vi "Parse Xml Recursively.vi"(7 "Parent":string, 8 "error in":errorcluster, 9 "XML File Path":path, 10 "DOM document in":refnum<k20>, 11 "VI Data":T1[](array[typedef])) -> (0 "error out":errorcluster, 3 "VI Data out":T1[](array[typedef]))   [LabVIEW 2020, in "VI Properties Editor.lvlib"]
uses:
  VI Properties Editor.lvlib
  CTLs/XPath Get Attribute.ctl
  <vilib>/picture/picture.llb/imagedata.ctl
  CTLs/VI Properties.ctl
  CTLs/Control Properties.ctl
  CTLs/VI Data.ctl
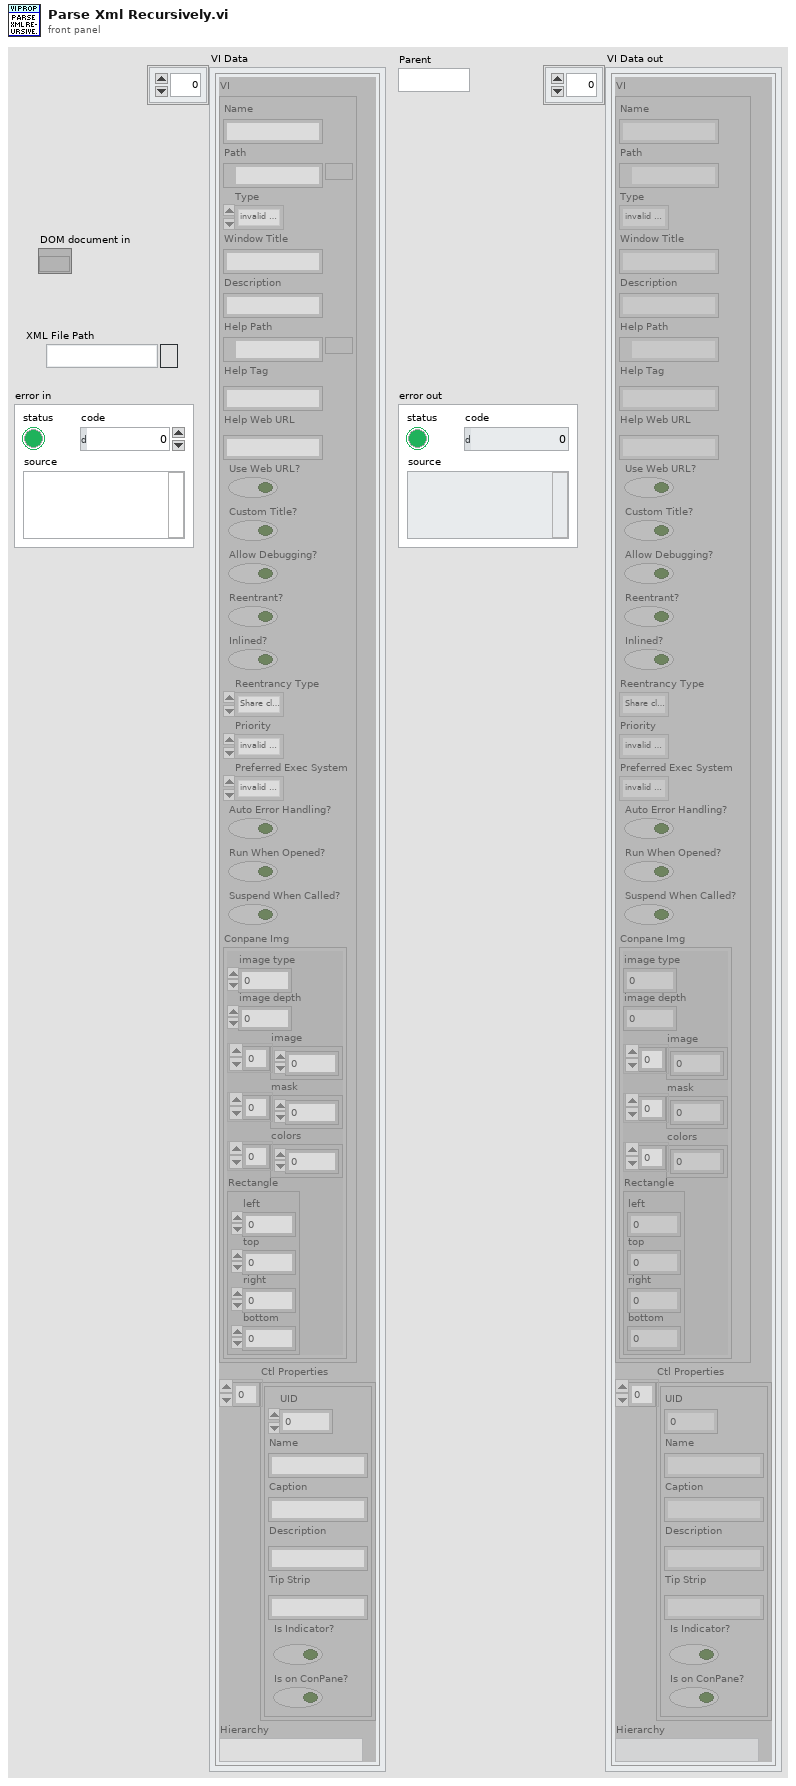
[diagram p1: front panel]
types:
  T1 = typedef "VI Properties Editor.lvlib/VI Data.ctl" = cluster{"VI":T2, "Ctl Properties":T4[], "Hierarchy":string}
  T2 = typedef "VI Properties Editor.lvlib/VI Properties.ctl" = cluster{"Name":string, "Path":path, "Type":enum32{"invalid VI type", "Standard VI", "Control VI", "Global VI", "Polymorphic VI", "Configuration VI", "SubSystem", "Facade VI", "Method VI", "Statechart Diagram VI"}, "Window Title":string, "Description":string, "Help Path":path, "Help Tag":string, "Help Web URL":string, "Use Web URL?":bool, "Custom Title?":bool, "Allow Debugging?":bool, "Reentrant?":bool, "Inlined?":bool, "Reentrancy Type":enum16{"Share clones between instances", "Preallocate clone for each instance"}, "Priority":enum32{"invalid priority", "background priority", "normal priority", "above normal priority", "high priority", "time critical priority", "subroutine"}, "Preferred Exec System":enum32{"invalid execution system", "user interface", "standard", "instrument i/o", "data acquisition", "other 1", "other 2", "same as caller"}, "Auto Error Handling?":bool, "Run When Opened?":bool, "Suspend When Called?":bool, "Conpane Img":T3}
  T3 = typedef "imagedata.ctl" = cluster{"image type":i32, "image depth":i32, "image":u8[], "mask":u8[], "colors":u32[], "Rectangle":cluster{"left":i16, "top":i16, "right":i16, "bottom":i16}}
  T4 = typedef "VI Properties Editor.lvlib/Control Properties.ctl" = cluster{"UID":i32, "Name":string, "Caption":string, "Description":string, "Tip Strip":string, "Is Indicator?":bool, "Is on ConPane?":bool}
  T5 = typedef "VI Properties Editor.lvlib/XPath Get Attribute.ctl" = enum16{"Item[@Type='VI']/@URL", "Item[@Type='LVClass']/@URL", "Item[@Type='Library']/@URL", "@Name"}
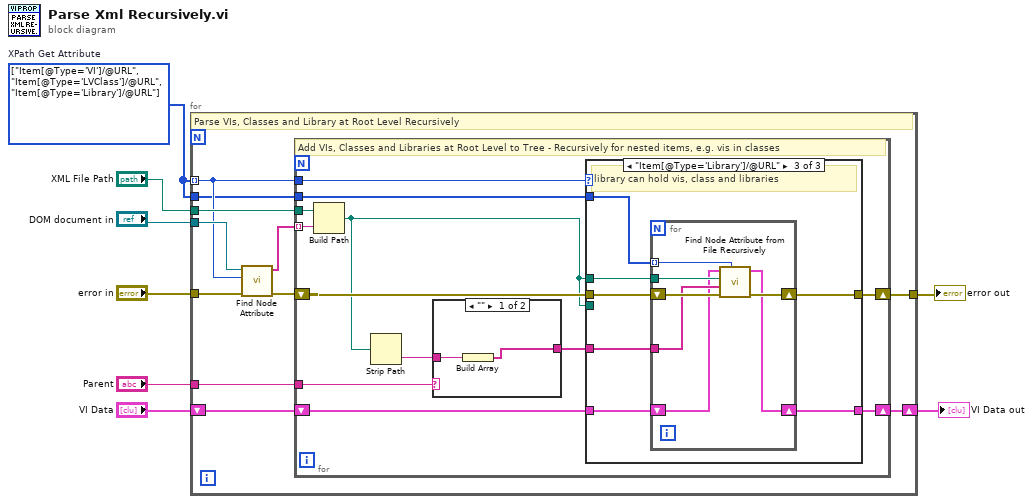
[diagram p0: block diagram]
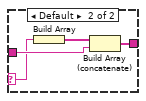
[diagram p2: hidden frame]
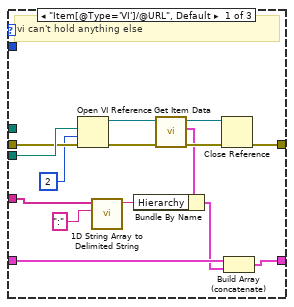
[diagram p3: hidden frame]
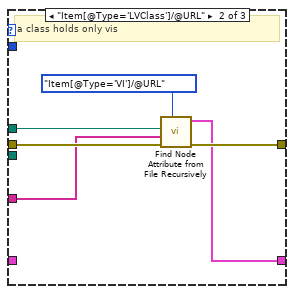
[diagram p4: hidden frame]
diagram:
  w5 = T5[] [enum."Item[@Type='VI']/@URL", enum."Item[@Type='LVClass']/@URL", enum."Item[@Type='Library']/@URL"] items=["Item[@Type='VI']/@URL", "Item[@Type='LVClass']/@URL", "Item[@Type='Library']/@URL", "@Name"]  # XPath Get Attribute
  n1 = for {
    tunnel: "XML File Path" -> [w18]
    tunnel: [w17] -> w6
    tunnel: "DOM document in" -> [w15]
    tunnel: "error in" -> [w14]
    tunnel: "Parent" -> [w13]
    shift-right: [w11] -> w1
    shift-left: "VI Data" -> [w12]
    tunnel: w5 -> [w10] mode=indexing
    tunnel: w5 -> [w9]
    # "Parse VIs, Classes and Library at Root Level Recursively"
    n2 = call "Find Node Attribute.vi"("error in"=w14, "XPath"=w10, "Node"=w15) -> ("error out"=w16:errorcluster, "Attribute"=w19:string[])  [unwired: 7 in]
    n3 = for {
      shift-right: [w31] -> w17
      shift-left: w16 -> [w27]
      tunnel: w10 -> [w28]
      tunnel: w18 -> [w29]
      tunnel: w19 -> [w30] mode=indexing
      tunnel: w13 -> [w24]
      shift-right: [w21] -> w11
      shift-left: w12 -> [w20]
      tunnel: w9 -> [w22]
      # "Add VIs, Classes and Libraries at Root Level to Tree - Recursively for nested items, e.g. vis in classes"
      n4 = Build Path(base path=w29, name or relative path=w30) -> (appended path=w23:path)
      n5 = Strip Path(path=w23) -> (name=w26:string)  [unwired: 1 out]
      n6 = case shown="\"\"" w24 {
        selector: w24 -> [_ w34]
        tunnel: w26 -> [w33 w37]
        tunnel: [w32 w36] -> w25
        frame "" {
          n7 = Build Array(w33) -> (w32:string[])
        }
        frame Default {
          n8 = Build Array(w34) -> (w35:string[])
          n9 = Build Array (concatenate)(w35, w37) -> (w36:string[])
        }
      }
      n10 = case shown="\"Item[@Type='Library']/@URL\"" w28 {
        tunnel: [w47 w58 w64] -> w31
        tunnel: w27 -> [w50 w57 w65]
        tunnel: w23 -> [_ w56 w63]
        tunnel: w25 -> [w43 w54 w62]
        tunnel: w23 -> [w51 _ _]
        tunnel: w22 -> [_ _ w61]
        tunnel: [w38 w53 w59] -> w21
        tunnel: w20 -> [w42 _ w60]
        frame "Item[@Type='VI']/@URL", Default {
          # "vi can't hold anything else"
          n11 = Open VI Reference(vi path=w51, options=2, error in (no error)=w50) -> (vi reference=w48:refnum<vi>, error out=w49:errorcluster)  [unwired: 3 in]
          n12 = call <vilib>:"1D String Array to Delimited String.vi"("delimiter"=":", "string array"=w43) -> ("delimited string"=w39:string)  [unwired: 9 in]
          n13 = call "Get Item Data.vi"("error in (no error)"=w49, "VI Ref"=w48) -> ("error out"=w52:errorcluster, "VI Data"=w41:T1, "VI Ref out"=w46:refnum<vi>)  [unwired: 7 in]
          n14 = Bundle By Name(cluster=w41, "Hierarchy"=w39) -> (w40:T1)
          n15 = Close Reference(reference=w46, error in (no error)=w52) -> (error out=w47:errorcluster)
          n16 = Build Array (concatenate)(w42, w40) -> (w38:T1[])
        }
        frame "Item[@Type='LVClass']/@URL" {
          # "a class holds only vis"
          n17 = call "Find Node Attribute from File Recursively.vi"("XPath"=XPath_Get_Attribute."Item[@Type='VI']/@URL", "error in"=w57, "Parent"=w54, "Path to XML document"=w56) -> ("error out"=w58:errorcluster, "VI Data out"=w53:T1[])  [unwired: 6 in]
        }
        frame "Item[@Type='Library']/@URL" {
          # "library can hold vis, class and libraries"
          n18 = for {
            tunnel: w63 -> [w70]
            tunnel: w61 -> [w69] mode=indexing
            tunnel: w62 -> [w68]
            shift-right: [w71] -> w64
            shift-left: w65 -> [w72]
            shift-right: [w66] -> w59
            shift-left: w60 -> [w67]
            n19 = call "Find Node Attribute from File Recursively.vi"("XPath"=w69, "error in"=w72, "Parent"=w68, "Path to XML document"=w70, "VI Data"=w67) -> ("error out"=w71:errorcluster, "VI Data out"=w66:T1[])  [unwired: 5 in]
          }
        }
      }
    }
  }
  "error out" <- w6
  "VI Data out" <- w1
